vi "Convert WGS84 to distance.vi"(6 "Lat2(dd)":dbl format="%.6f", 7 "Lat1(dd)":dbl format="%.6f", 8 "Lon2(dd)":dbl format="%.6f", 9 "Lon1(dd)":dbl format="%.6f") -> (0 "Heading":dbl format="%.2f", 1 "Delta Long(ft)":dbl format="%.2f", 2 "Delta Lat(ft)":dbl format="%.2f", 3 "Distance(feet)":dbl format="%.6f", 4 "Delta Lat(dd)":dbl format="%.2f", 5 "Delta Long(dd)":dbl format="%.2f")   [LabVIEW 2015]
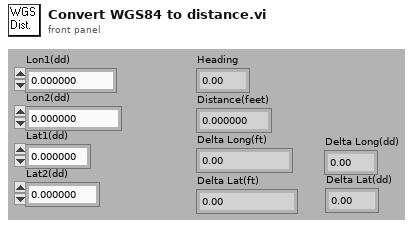
[diagram p1: front panel]
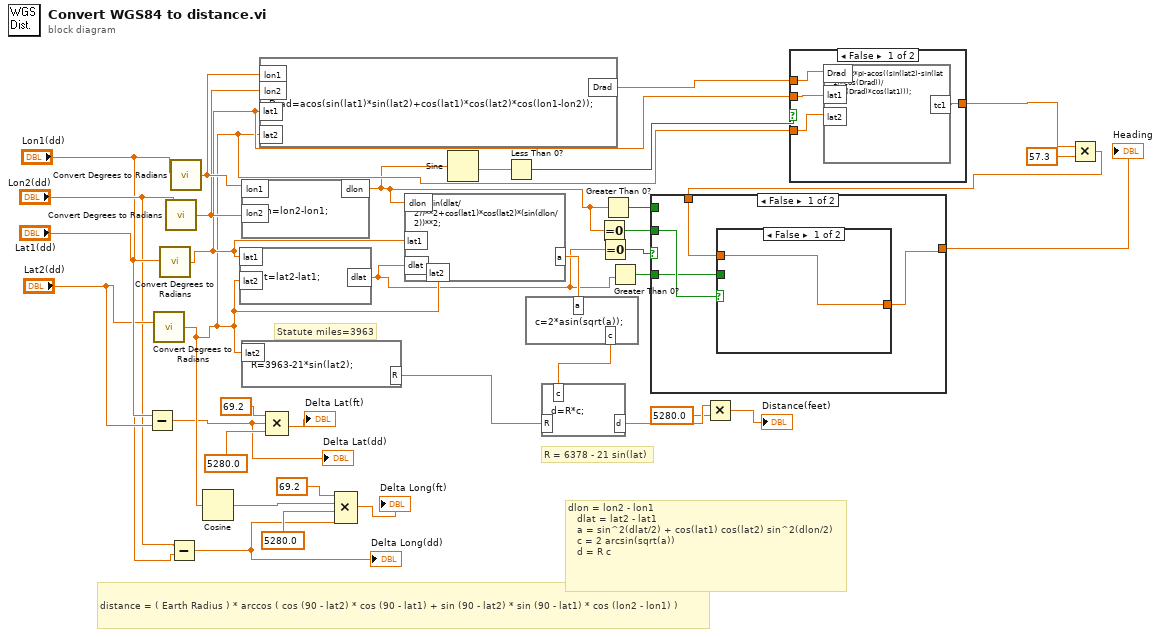
[diagram p0: block diagram]
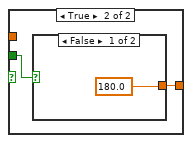
[diagram p2: hidden frame]
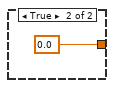
[diagram p3: hidden frame]
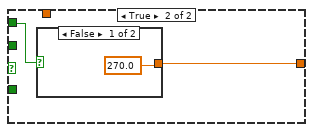
[diagram p4: hidden frame]
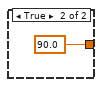
[diagram p5: hidden frame]
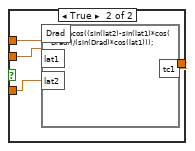
[diagram p6: hidden frame]
diagram:
  # "Statute miles=3963"
  # "distance = ( Earth Radius ) * arccos ( cos (90 - lat2) * cos (90 - lat1) + sin (90 - lat2) * sin (90 - lat1) * cos (lon2 - lon1) )"
  # "R = 6378 - 21 sin(lat)"
  # "dlon = lon2 - lon1\n   dlat = lat2 - lat1\n   a = sin^2(dlat/2) + cos(lat1) cos(lat2) sin^2(dlon/2)\n   c = 2 arcsin(sqrt(a))\n   d = R c"
  n1 = Subtract(x="Lat1(dd)", y="Lat2(dd)") -> (x-y=w11:dbl)
  "Delta Lat(dd)" <- w11
  n2 = call "Convert Degrees to Radians.vi"("Deg"="Lat2(dd)") -> ("rad"=w15:dbl)
  n3 = call "Convert Degrees to Radians.vi"("Deg"="Lat1(dd)") -> ("rad"=w20:dbl)
  n4 = call "Convert Degrees to Radians.vi"("Deg"="Lon2(dd)") -> ("rad"=w25:dbl)
  n5 = Subtract(x="Lon2(dd)", y="Lon1(dd)") -> (x-y=w10:dbl)
  "Delta Long(dd)" <- w10
  n6 = call "Convert Degrees to Radians.vi"("Deg"="Lon1(dd)") -> ("rad"=w26:dbl)
  n7 = Cosine(x=w15) -> (cos(x)=w14:dbl)
  n8 = formula code="dlat=lat2-lat1;"("lat1"=w20, "lat2"=w15) -> ("dlat"=w5:dbl)
  n9 = formula code="dlon=lon2-lon1;"("lon1"=w26, "lon2"=w25) -> ("dlon"=w7:dbl)
  n10 = formula code="R=3963-21*sin(lat2);"("lat2"=w15) -> ("R"=w34:dbl)
  n11 = formula code="Drad=acos(sin(lat1)*sin(lat2)+cos(lat1)*cos(lat2)*cos(lon1-lon2));"("lon1"=w26, "lon2"=w25, "lat1"=w20, "lat2"=w15) -> ("Drad"=w21:dbl)
  n12 = Compound Arithmetic op=MULTIPLY(69.2 ("Input"), w11, 5280.0 ("y")) -> (→"Delta Lat(ft)":dbl)
  n13 = Compound Arithmetic op=MULTIPLY(69.2 ("Input"), w14, 5280.0 ("y"), w10) -> (→"Delta Long(ft)":dbl)
  n14 = formula code="a=(sin(dlat/2))**2+cos(lat1)*cos(lat2)*(sin(dlon/2))**2;"("dlon"=w7, "dlat"=w5, "lat1"=w20, "lat2"=w15) -> ("a"=w36:dbl)
  n15 = Sine(x=w7) -> (sin(x)=w24:dbl)
  n16 = Less Than 0?(x=w24) -> (x < 0?=w22:bool)
  n17 = formula code="c=2*asin(sqrt(a));"("a"=w36) -> ("c"=w35:dbl)
  n18 = formula code="d=R*c;"("c"=w35, "R"=w34) -> ("d"=w33:dbl)
  n19 = Equal To 0?(x=w7) -> (x = 0?=w6:bool)
  n20 = Equal To 0?(x=w5) -> (x = 0?=w9:bool)
  n21 = Greater Than 0?(x=w7) -> (x > 0?=w8:bool)
  n22 = Greater Than 0?(x=w5) -> (x > 0?=w4:bool)
  n23 = Multiply(x=w33, y=5280.0) -> (x*y=→"Distance(feet)":dbl)
  n24 = case shown="False" w22 {
    tunnel: w20 -> [w39 w44]
    tunnel: w15 -> [w38 w43]
    tunnel: w21 -> [w40 w42]
    tunnel: [w37 w41] -> w3
    frame False {
      n25 = formula code="tc1=2*pi-acos((sin(lat2)-sin(lat1)*cos(Drad))/(sin(Drad)*cos(lat1)));"("lat1"=w39, "lat2"=w38, "Drad"=w40) -> ("tc1"=w37:dbl)
    }
    frame True {
      n26 = formula code="tc1=acos((sin(lat2)-sin(lat1)*cos(Drad))/(sin(Drad)*cos(lat1)));"("lat1"=w44, "lat2"=w43, "Drad"=w42) -> ("tc1"=w41:dbl)
    }
  }
  n27 = Multiply(x=w3, y=57.3) -> (x*y=w2:dbl)
  n28 = case shown="False" w9 {
    tunnel: [w46 w55] -> w1
    tunnel: w8 -> [_ w54]
    tunnel: w6 -> [w48 _]
    tunnel: w4 -> [w47 _]
    tunnel: w2 -> [w45 _]
    frame False {
      n29 = case shown="False" w48 {
        tunnel: w47 -> [_ w51]
        tunnel: [w49 w50] -> w46
        tunnel: w45 -> [w49 _]
        frame False {
        }
        frame True {
          n30 = case shown="False" w51 {
            tunnel: [180.0 0.0] -> w50
            frame False {
            }
            frame True {
            }
          }
        }
      }
    }
    frame True {
      n31 = case shown="False" w54 {
        tunnel: [270.0 90.0] -> w55
        frame False {
        }
        frame True {
        }
      }
    }
  }
  "Heading" <- w1
